vi "GetEvents.vi"(8 "error in (no error)":errorcluster, 11 "CameraSim in":refnum<class "CameraI2COUSB.lvclass">) -> (0 "error out":errorcluster, 2 "Events":T1, 3 "CameraSim out":refnum<class "CameraI2COUSB.lvclass">)   [LabVIEW 2020, in "Camera.lvlib" / "CameraI2COUSB.lvclass"]
doc: "Return events generates from camera"
uses:
  CameraI2COUSB.lvclass
  ICamera/ICamera/TypeDef/Events.ctl
  ICamera/ICamera/TypeDef/StreamDataEvent.ctl
  CameraI2COUSB.lvclass/CameraI2COUSB.ctl
  ICamera/ICamera/ICamera.lvclass
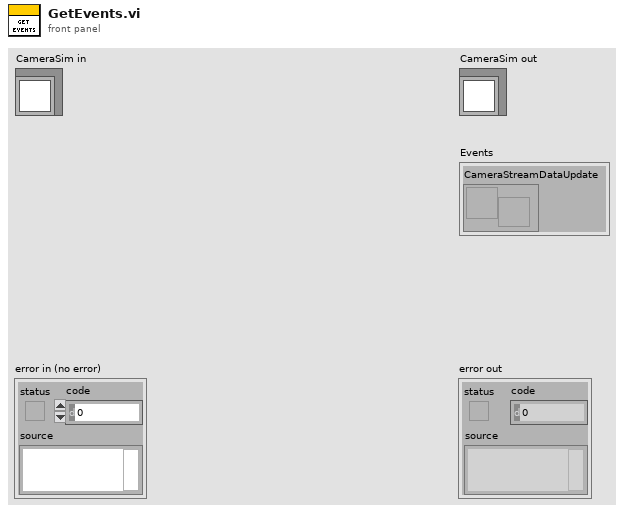
[diagram p1: front panel]
types:
  T1 = typedef "ICamera.lvlib/ICamera.lvclass/Events.ctl" = cluster{"CameraStreamDataUpdate":T2}
  T2 = typedef "ICamera.lvlib/ICamera.lvclass/StreamDataEvent.ctl" = refnum<user-event>
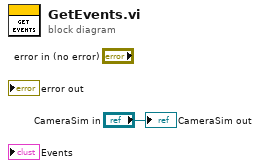
[diagram p0: block diagram]
diagram:
  "CameraSim out" <- "CameraSim in"
